vi "points2length.vi"(4 "z1":dbl, 5 "z0":dbl, 6 "y1":dbl, 7 "y0":dbl, 8 "x1":dbl, 11 "x0":dbl) -> (0 "dz":dbl, 1 "dy":dbl, 2 "dx":dbl, 3 "Length":dbl)   [LabVIEW 2023]
doc: "Calculates the length difference between two points (x0,y0,z0),(x1,y1,z1)."
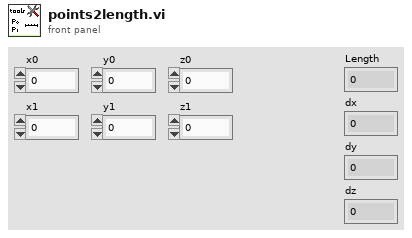
[diagram p1: front panel]
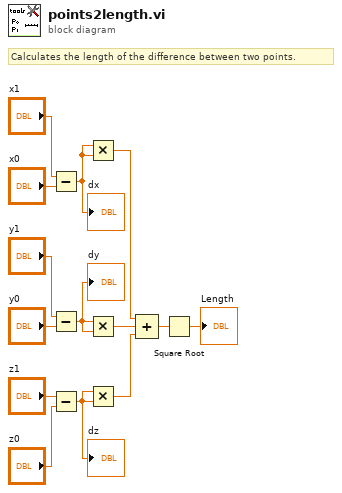
[diagram p0: block diagram]
diagram:
  # "Calculates the length of the difference between two points."
  n1 = Subtract(x="x1", y="x0") -> (x-y=w3:dbl)
  "dx" <- w3
  n2 = Subtract(x="y1", y="y0") -> (x-y=w2:dbl)
  "dy" <- w2
  n3 = Subtract(x="z1", y="z0") -> (x-y=w1:dbl)
  "dz" <- w1
  n4 = Multiply(x=w3, y=w3) -> (x*y=w9:dbl)
  n5 = Multiply(x=w2, y=w2) -> (x*y=w8:dbl)
  n6 = Multiply(x=w1, y=w1) -> (x*y=w4:dbl)
  n7 = Compound Arithmetic op=ADD(w9, w8, w4) -> (w10:dbl)
  n8 = Square Root(x=w10) -> (sqrt(x)=→"Length":dbl)
